vi "LED Intensity Picker [RT].vi"() -> ()   [LabVIEW 2016]
uses:
  <vilib>/Platform/TimedLoop/XDataNode/timing_clust.ctl
  <vilib>/Platform/TimedLoop/XDataNode/nitl_modes.ctl
  <vilib>/Platform/TimedLoop/XDataNode/wakeup.ctl
  <vilib>/FPGAPlugInAG/sbRIO-9637/niLvFpga_Open_sbRIO-9637.vi
  <vilib>/rvi/interface/common/dynamic/niFpgaDynamicAddResources.vi
  <vilib>/Utility/error.llb/Error Cluster From Error Code.vi
  <vilib>/rvi/errors/niLvFpgaAdjustHostInterfaceError.vi
  <vilib>/FPGAPlugInAG/Dynamic/niLvFpga_Close_Dynamic.vi
  <vilib>/Platform/TimedLoop/XDataNode/XDataNode.xnode
  <vilib>/rvi/interface/nirviOpenFPGA/nirviOpenFPGA.xnode
  FPGA Bitfiles/Exercise1_FPGATarget_LEDPWM[FPGA]_gnxrx5kCNbg.lvbitx
  <vilib>/rvi/interface/nirviReadWriteControl/nirviReadWriteControl.xnode
  <vilib>/rvi/interface/nirviCloseFPGA/nirviCloseFPGA.xnode
  <vilib>/Platform/TimedLoop/XDataNode/XDNodeRunTimeDep.lvlib
  NiFpgaLv.dll
  <vilib>/rvi/interface/Simulation/niFpgaSimulationCallBeginRW.vi
panel:
  in  "Pulse Period (s)":dbl(slide)=2.0 min=0.01 scale=0.0..6.0
  in  "Pulse LEDs":bool
  out "LED1":u32(colorbox)=16711680
  in  "LED1 Intensity (%)":dbl(slide)=100.0 scale=0.0..100.0 scale format="%#_6g%"
  out "LED0":u32(colorbox)=16711680
  in  "LED0 Intensity (%)":dbl(slide)=100.0 scale=0.0..100.0 scale format="%#_6g%"
  in  "Stop":bool
  # "LED1 Intensity"
  # "LED0 Intensity"
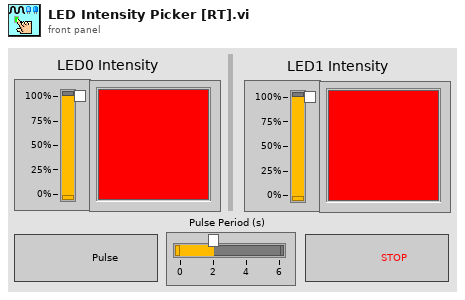
[diagram p1: front panel]
types:
  T1 = typedef "XDNodeRunTimeDep.lvlib/timing_clust.ctl" = cluster{"Expected End [f-1]":u64, "Actual End [f-1]":u64, "Finished Late? [f-1]":bool, "Expected End [i-1]":u64, "Actual End [i-1]":u64, "Finished Late? [i-1]":bool, "Expected Start [i]":u64, "Actual Start [i]":u64, "Expected Start [f]":u64, "Actual Start [f]":u64, "Source Name":string, "Structure Name":string, "Period":i64, "Deadline":i64, "Offset":i64, "Start":i64, "Priority":i32, "Timeout":i32, "Mode":T2, "Wakeup Reason":T3, "Error":errorcluster, "Source Type":string, "Secondary Source Type":string, "Global End Time":u64, "Global Start Time":u64, "Frame Duration":u64, "Iteration Duration":u64, "Assigned CPU":i32, "I/O Scan Engine Mode":u32}
  T2 = typedef "XDNodeRunTimeDep.lvlib/nitl_modes.ctl" = enum32{"No Change", "Process missed periods, maintain original phase", "Discard missed periods, maintain original phase", "Process missed periods, ignore original phase", "Discard missed periods, ignore original phase"}
  T3 = typedef "XDNodeRunTimeDep.lvlib/wakeup.ctl" = enum32{"Normal", "Aborted", "Asynchronous wakeup", "Timing source error", "Timed loop error", "Timeout"}
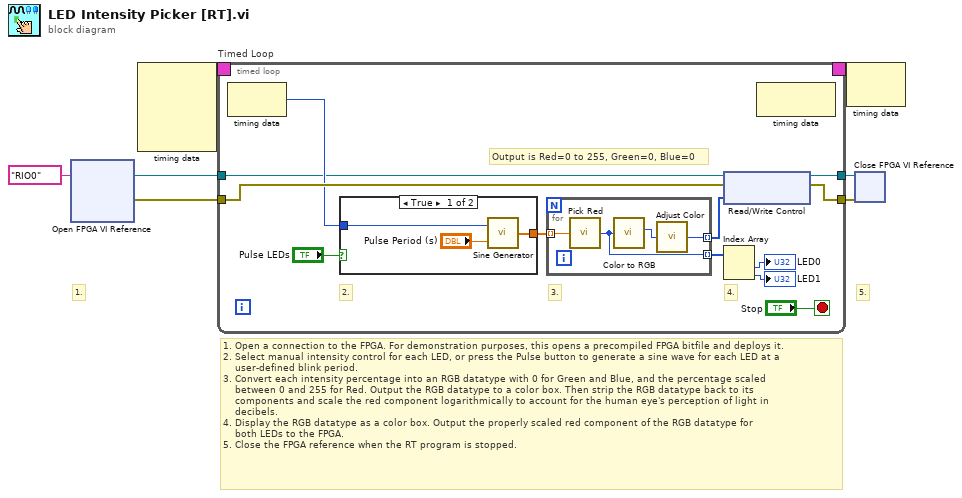
[diagram p0: block diagram]
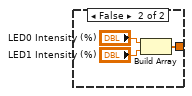
[diagram p2: hidden frame]
diagram:
  # "5."
  # "1. Open a connection to the FPGA. For demonstration purposes, this opens a precompiled FPGA bitfile and deploys it.\n2. Select manual intensity control for each LED, or press the Pulse button to generate a sine wave for each LED at a \n    user-defined blink period.\n3. Convert each intensity percentage into an RGB datatype with 0 for Green and Blue, and the percentage scaled\n    between 0 and 255 for Red. Output the RGB datatype to a color box. Then strip the RGB datatype back to its \n    components and scale the red component logarithmically to account for the human eye's perception of light in\n    decibels.\n4. Display the RGB datatype as a color box. Output the properly scaled red component of the RGB datatype for\n    both LEDs to the FPGA.\n5. Close the FPGA reference when the RT program is stopped."
  # "1."
  n1 = xnode "Open FPGA VI Reference"("resource name"=tag "RIO0") -> ("FPGA VI Reference Out"=w5:refnum<k20>, "error out"=w3:errorcluster)  [unwired: 1 in]
  n2 = node-c288() -> (w7:T1)  [unwired: 4 in]
  n3 = timed-loop "Timed Loop" {
    timing: w7 -> [_]
    timing-out: [_] -> w6
    tunnel: w5 -> [w8]
    tunnel: [w14] -> w4
    tunnel: w3 -> [w12]
    tunnel: [w11] -> w2
    stop <- "Stop" stop-if-true
    # "Output is Red=0 to 255, Green=0, Blue=0"
    # "4."
    # "3."
    # "2."
    n4 = node-c288() -> (w10:i64)  [unwired: 1 in]
    n5 = case shown="True" "Pulse LEDs" {
      tunnel: [w22 w23] -> w18
      tunnel: w10 -> [w20 _]
      frame True {
        n6 = call "Sine Generator.vi"("Blink Period (s)"="Pulse Period (s)", "Loop Rate (ms)"=w20) -> ("Intensity (%)"=w22:dbl[])
      }
      frame False {
        n7 = Build Array("LED0 Intensity (%)", "LED1 Intensity (%)") -> (w23:dbl[])
      }
    }
    n8 = for {
      tunnel: w18 -> [w29] mode=indexing
      tunnel: [w28] -> w17 mode=indexing
      tunnel: [w27] -> w13 mode=indexing
      n9 = call "Pick Red.vi"("Intensity (%)"=w29) -> ("Red Hue"=w28:u32)
      n10 = call <vilib>:"Color to RGB.vi"("Color"=w28) -> ("R"=w26:u8)  [unwired: 3 out]
      n11 = call "Adjust Color.vi"("Greyscale In"=w26) -> ("Greyscale Out"=w27:u8)
    }
    n12 = xnode "Read/Write Control"("FPGA VI Reference In"=w8, "error in"=w12, "LED Intensity"=w13) -> ("FPGA VI Reference Out"=w14:refnum<k20>, "error out"=w11:errorcluster)
    n13 = Index Array(array=w17) -> (element #1=→"LED0":u32, element #2=→"LED1":u32)  [unwired: 2 in]
    n14 = node-c288() -> ()  [unwired: 1 in, 1 out]
  }
  n15 = node-c288(w6) -> ()  [unwired: 1 out]
  n16 = xnode "Close FPGA VI Reference"("FPGA VI Reference In"=w4, "error in"=w2) -> ()  [unwired: 1 out]
